vi "Global 2.vi"() -> ()   [LabVIEW 2018]
panel:
  in  "UsePython":bool caption="Tank RF"
  out "Fit OK":bool
  in  "Fupper":dbl=213.2 format="%#_13g"
  in  "Flower":dbl=212.8 format="%#_13g"
  in  "AutoFreq":bool
  in  "Tune file":string="Tune2.csv"
  out "Beam ON":bool=TRUE
  in  "NMR Channel":i32=2 min=0 max=7 step=1
  in  "TEQ Comment":string="Unused"
  in  "Q Comment":string="Newest  213 MHz Q curve 5/2/18"
  in  "TEQ file":string="NMRave.csv"
  in  "Measurement":enum16{"TEQ", "POL", "QCV"}(ring)=enum."QCV"
  in  "Commentary":string="Start trying python Q curve subtraction"
  in  "Calib Constant":dbl=1000.0 min=0.0 max=1000.0 step=0.001 format="%_3f"
  out "File name":string="C:\\users\\Ptgroup\\Desktop\\rssmt\\data\\22\\QCV3830786383.csv"
  in  "IP Address":string="192.168.24.146"
  in  "Gain":enum16{"LOW", "HI", "MAX"}(ring)
  in  "COM Port #":refnum<visa-resource-name>="COM8"
  out "Peak center (MHz)":sgl=212.9519 format="%.3f"
  in  "Logoffset (V)":dbl min=-9.0 max=0.0 step=0.0005 format="%_5g"
  in  "Phase (V)":dbl=2.566 min=-0.4 max=10.7 step=0.0005 format="%_5g"
  in  "Real/Quad Q curve":bool=TRUE
  out "Temperature (C)":dbl(graph)=24.75
  out "+3V supply":dbl=3.265 format="%_4g"
  out "Temp (C)":dbl=24.75 format="%_4g"
  in  "RemovePed":bool=TRUE
  in  "IF / LOG Det":bool=TRUE
  in  "Q curve file":string="QCV3608133393.csv"
  in  "AutoTune":bool
  out "RF OK":bool=TRUE
  out "Peak area (mV-MHz)":sgl=0.727321 format="%.3e"
  in  "Gauss Fit":bool
  out "NMR Graph + Fit":cluster{cluster{dbl, "Numeric":dbl}[]}[](graph)=[{[{224.27, "Numeric"=0.0}, {224.2705, "Numeric"=0.0}, {224.27100000000002, "Numeric"=0.0}, {224.2715, "Numeric"=0.0}, {224.27200000000002, "Numeric"=0.0}, {224.2725, "Numeric"=0.0}, {224.273, "Numeric"=0.0}, {224.2735, "Numeric"=0.0}, {224.274, "Numeric"=0.0}, {224.27450000000002, "Numeric"=0.0}, {224.275, "Numeric"=0.0}, {224.27550000000002, "Numeric"=0.0}, {224.276, "Numeric"=0.0}, {224.2765, "Numeric"=0.0}, {224.27700000000002, "Numeric"=0.0}, {224.2775, "Numeric"=0.0}, {224.27800000000002, "Numeric"=0.0}, {224.2785, "Numeric"=0.0}, {224.279, "Numeric"=0.0}, {224.2795, "Numeric"=0.0}, {224.28, "Numeric"=0.0}, {224.28050000000002, "Numeric"=0.0}, {224.281, "Numeric"=0.0}, {224.28150000000002, "Numeric"=0.0}, {224.282, "Numeric"=0.0}, {224.2825, "Numeric"=0.0}, {224.28300000000002, "Numeric"=0.0}, {224.2835, "Numeric"=0.0}, {224.28400000000002, "Numeric"=0.0}, {224.2845, "Numeric"=0.0}, {224.285, "Numeric"=0.0}, {224.2855, "Numeric"=0.0}, {224.286, "Numeric"=0.0}, {224.28650000000002, "Numeric"=0.0}, {224.287, "Numeric"=0.0}, {224.28750000000002, "Numeric"=0.0}, {224.288, "Numeric"=0.0}, {224.2885, "Numeric"=0.0}, {224.28900000000002, "Numeric"=0.0}, {224.2895, "Numeric"=0.0}, {224.29000000000002, "Numeric"=0.0}, {224.2905, "Numeric"=0.0}, {224.291, "Numeric"=0.0}, {224.2915, "Numeric"=0.0}, {224.292, "Numeric"=0.0}, {224.29250000000002, "Numeric"=0.0}, {224.293, "Numeric"=0.0}, {224.29350000000002, "Numeric"=0.0}, {224.294, "Numeric"=0.0}, {224.2945, "Numeric"=0.0}, {224.29500000000002, "Numeric"=0.0}, {224.2955, "Numeric"=0.0}, {224.29600000000002, "Numeric"=0.0}, {224.2965, "Numeric"=0.0}, {224.297, "Numeric"=0.0}, {224.2975, "Numeric"=0.0}, {224.298, "Numeric"=0.0}, {224.29850000000002, "Numeric"=0.0}, {224.299, "Numeric"=0.0}, {224.2995, "Numeric"=0.0}, {224.3, "Numeric"=0.0}, {224.3005, "Numeric"=0.0}, {224.30100000000002, "Numeric"=0.0}, {224.3015, "Numeric"=0.0}, {224.30200000000002, "Numeric"=0.0}, {224.3025, "Numeric"=0.0}, {224.303, "Numeric"=0.0}, {224.3035, "Numeric"=0.0}, {224.304, "Numeric"=0.0}, {224.30450000000002, "Numeric"=0.0}, {224.305, "Numeric"=0.0}, {224.3055, "Numeric"=0.0}, {224.306, "Numeric"=0.0}, {224.3065, "Numeric"=0.0}, {224.30700000000002, "Numeric"=0.0}, {224.3075, "Numeric"=0.0}, {224.30800000000002, "Numeric"=0.0}, {224.3085, "Numeric"=0.0}, {224.309, "Numeric"=0.0}, {224.3095, "Numeric"=0.0}, {224.31, "Numeric"=0.0}, {224.31050000000002, "Numeric"=0.0}, {224.311, "Numeric"=0.0}, {224.3115, "Numeric"=0.0}, {224.312, "Numeric"=0.0}, {224.3125, "Numeric"=0.0}, {224.31300000000002, "Numeric"=0.0}, {224.3135, "Numeric"=0.0}, {224.31400000000002, "Numeric"=0.0}, {224.3145, "Numeric"=0.0}, {224.315, "Numeric"=0.0}, {224.31550000000001, "Numeric"=0.0}, {224.316, "Numeric"=0.0}, {224.31650000000002, "Numeric"=0.0}, {224.317, "Numeric"=0.0}, {224.3175, "Numeric"=0.0}, {224.318, "Numeric"=0.0}, {224.3185, "Numeric"=0.0}, {224.31900000000002, "Numeric"=0.0}, {224.3195, "Numeric"=0.0}, {224.32, "Numeric"=0.0}, {224.3205, "Numeric"=0.0}, {224.321, "Numeric"=0.0}, {224.32150000000001, "Numeric"=0.0}, {224.322, "Numeric"=0.0}, {224.32250000000002, "Numeric"=0.0}, {224.323, "Numeric"=0.0}, {224.3235, "Numeric"=0.0}, {224.324, "Numeric"=0.0}, {224.3245, "Numeric"=0.0}, {224.32500000000002, "Numeric"=0.0}, {224.3255, "Numeric"=0.0}, {224.326, "Numeric"=0.0}, {224.3265, "Numeric"=0.0}, {224.327, "Numeric"=0.0}, {224.32750000000001, "Numeric"=0.0}, {224.328, "Numeric"=0.0}, {224.32850000000002, "Numeric"=0.0}, {224.329, "Numeric"=0.0}, {224.3295, "Numeric"=0.0}, {224.33, "Numeric"=0.0}, {224.3305, "Numeric"=0.0}, {224.33100000000002, "Numeric"=0.0}, {224.3315, "Numeric"=0.0}, {224.332, "Numeric"=0.0}, {224.3325, "Numeric"=0.0}, {224.333, "Numeric"=0.0}, {224.33350000000002, "Numeric"=0.0}, {224.334, "Numeric"=0.0}, {224.33450000000002, "Numeric"=0.0}, {224.335, "Numeric"=0.0}, {224.3355, "Numeric"=0.0}, {224.336, "Numeric"=0.0}, {224.3365, "Numeric"=0.0}, {224.33700000000002, "Numeric"=0.0}, {224.3375, "Numeric"=0.0}, {224.338, "Numeric"=0.0}, {224.3385, "Numeric"=0.0}, {224.339, "Numeric"=0.0}, {224.33950000000002, "Numeric"=0.0}, {224.34, "Numeric"=0.0}, {224.34050000000002, "Numeric"=0.0}, {224.341, "Numeric"=0.0}, {224.3415, "Numeric"=0.0}, {224.342, "Numeric"=0.0}, {224.3425, "Numeric"=0.0}, {224.34300000000002, "Numeric"=0.0}, {224.3435, "Numeric"=0.0}, {224.344, "Numeric"=0.0}, {224.3445, "Numeric"=0.0}, {224.345, "Numeric"=0.0}, {224.34550000000002, "Numeric"=0.0}, {224.346, "Numeric"=0.0}, {224.3465, "Numeric"=0.0}, {224.347, "Numeric"=0.0}, {224.3475, "Numeric"=0.0}, {224.348, "Numeric"=0.0}, {224.3485, "Numeric"=0.0}, {224.34900000000002, "Numeric"=0.0}, {224.3495, "Numeric"=0.0}, {224.35, "Numeric"=0.0}, {224.3505, "Numeric"=0.0}, {224.351, "Numeric"=0.0}, {224.35150000000002, "Numeric"=0.0}, {224.352, "Numeric"=0.0}, {224.3525, "Numeric"=0.0}, {224.353, "Numeric"=0.0}, {224.3535, "Numeric"=0.0}, {224.354, "Numeric"=0.0}, {224.3545, "Numeric"=0.0}, {224.35500000000002, "Numeric"=0.0}, {224.3555, "Numeric"=0.0}, {224.356, "Numeric"=0.0}, {224.3565, "Numeric"=0.0}, {224.357, "Numeric"=0.0}, {224.35750000000002, "Numeric"=0.0}, {224.358, "Numeric"=0.0}, {224.3585, "Numeric"=0.0}, {224.359, "Numeric"=0.0}, {224.3595, "Numeric"=0.0}, {224.36, "Numeric"=0.0}, {224.3605, "Numeric"=0.0}, {224.36100000000002, "Numeric"=0.0}, {224.3615, "Numeric"=0.0}, {224.362, "Numeric"=0.0}, {224.3625, "Numeric"=0.0}, {224.363, "Numeric"=0.0}, {224.36350000000002, "Numeric"=0.0}, {224.364, "Numeric"=0.0}, {224.3645, "Numeric"=0.0}, {224.365, "Numeric"=0.0}, {224.3655, "Numeric"=0.0}, {224.366, "Numeric"=0.0}, {224.3665, "Numeric"=0.0}, {224.36700000000002, "Numeric"=0.0}, {224.3675, "Numeric"=0.0}, {224.368, "Numeric"=0.0}, {224.3685, "Numeric"=0.0}, {224.369, "Numeric"=0.0}, {224.36950000000002, "Numeric"=0.0}, {224.37, "Numeric"=0.0}, {224.3705, "Numeric"=0.0}, {224.371, "Numeric"=0.0}, {224.3715, "Numeric"=0.0}, {224.372, "Numeric"=0.0}, {224.3725, "Numeric"=0.0}, {224.373, "Numeric"=0.0}, {224.3735, "Numeric"=0.0}, {224.374, "Numeric"=0.0}, {224.3745, "Numeric"=0.0}, {224.375, "Numeric"=0.0}, {224.37550000000002, "Numeric"=0.0}, {224.376, "Numeric"=0.0}, {224.3765, "Numeric"=0.0}, {224.377, "Numeric"=0.0}, {224.3775, "Numeric"=0.0}, {224.37800000000001, "Numeric"=0.0}, {224.3785, "Numeric"=0.0}, {224.379, "Numeric"=0.0}, {224.3795, "Numeric"=0.0}, {224.38, "Numeric"=0.0}, {224.3805, "Numeric"=0.0}, {224.381, "Numeric"=0.0}, {224.38150000000002, "Numeric"=0.0}, {224.382, "Numeric"=0.0}, {224.3825, "Numeric"=0.0}, {224.383, "Numeric"=0.0}, {224.3835, "Numeric"=0.0}, {224.38400000000001, "Numeric"=0.0}, {224.3845, "Numeric"=0.0}, {224.385, "Numeric"=0.0}, {224.3855, "Numeric"=0.0}, {224.386, "Numeric"=0.0}, {224.3865, "Numeric"=0.0}, {224.387, "Numeric"=0.0}, {224.38750000000002, "Numeric"=0.0}, {224.388, "Numeric"=0.0}, {224.3885, "Numeric"=0.0}, {224.389, "Numeric"=0.0}, {224.3895, "Numeric"=0.0}, {224.39000000000001, "Numeric"=0.0}, {224.3905, "Numeric"=0.0}, {224.391, "Numeric"=0.0}, {224.3915, "Numeric"=0.0}, {224.392, "Numeric"=0.0}, {224.3925, "Numeric"=0.0}, {224.393, "Numeric"=0.0}, {224.39350000000002, "Numeric"=0.0}, {224.394, "Numeric"=0.0}, {224.3945, "Numeric"=0.0}, {224.395, "Numeric"=0.0}, {224.3955, "Numeric"=0.0}, {224.39600000000002, "Numeric"=0.0}, {224.3965, "Numeric"=0.0}, {224.397, "Numeric"=0.0}, {224.3975, "Numeric"=0.0}, {224.398, "Numeric"=0.0}, {224.3985, "Numeric"=0.0}, {224.399, "Numeric"=0.0}, {224.3995, "Numeric"=0.0}, {224.4, "Numeric"=0.0}, {224.4005, "Numeric"=0.0}, {224.401, "Numeric"=0.0}, {224.4015, "Numeric"=0.0}, {224.40200000000002, "Numeric"=0.0}, {224.4025, "Numeric"=0.0}, {224.403, "Numeric"=0.0}, {224.4035, "Numeric"=0.0}, {224.404, "Numeric"=0.0}, {224.4045, "Numeric"=0.0}, {224.405, "Numeric"=0.0}, {224.4055, "Numeric"=0.0}, {224.406, "Numeric"=0.0}, {224.4065, "Numeric"=0.0}, {224.407, "Numeric"=0.0}, {224.4075, "Numeric"=0.0}, {224.40800000000002, "Numeric"=0.0}, {224.4085, "Numeric"=0.0}, {224.409, "Numeric"=0.0}, {224.4095, "Numeric"=0.0}, {224.41, "Numeric"=0.0}, {224.4105, "Numeric"=0.0}, {224.411, "Numeric"=0.0}, {224.4115, "Numeric"=0.0}, {224.412, "Numeric"=0.0}, {224.4125, "Numeric"=0.0}, {224.413, "Numeric"=0.0}, {224.4135, "Numeric"=0.0}, {224.41400000000002, "Numeric"=0.0}, {224.4145, "Numeric"=0.0}, {224.415, "Numeric"=0.0}, {224.4155, "Numeric"=0.0}, {224.416, "Numeric"=0.0}, {224.4165, "Numeric"=0.0}, {224.417, "Numeric"=0.0}, {224.4175, "Numeric"=0.0}, {224.418, "Numeric"=0.0}, {224.4185, "Numeric"=0.0}, {224.419, "Numeric"=0.0}, {224.4195, "Numeric"=0.0}, {224.42000000000002, "Numeric"=0.0}, {224.4205, "Numeric"=0.0}, {224.421, "Numeric"=0.0}, {224.4215, "Numeric"=0.0}, {224.422, "Numeric"=0.0}, {224.4225, "Numeric"=0.0}, {224.423, "Numeric"=0.0}, {224.4235, "Numeric"=0.0}, {224.424, "Numeric"=0.0}, {224.4245, "Numeric"=0.0}, {224.425, "Numeric"=0.0}, {224.4255, "Numeric"=0.0}, {224.426, "Numeric"=0.0}, {224.4265, "Numeric"=0.0}, {224.427, "Numeric"=0.0}, {224.4275, "Numeric"=0.0}, {224.428, "Numeric"=0.0}, {224.4285, "Numeric"=0.0}, {224.429, "Numeric"=0.0}, {224.4295, "Numeric"=0.0}, {224.43, "Numeric"=0.0}, {224.4305, "Numeric"=0.0}, {224.431, "Numeric"=0.0}, {224.4315, "Numeric"=0.0}, {224.432, "Numeric"=0.0}, {224.4325, "Numeric"=0.0}, {224.433, "Numeric"=0.0}, {224.4335, "Numeric"=0.0}, {224.434, "Numeric"=0.0}, {224.4345, "Numeric"=0.0}, {224.435, "Numeric"=0.0}, {224.4355, "Numeric"=0.0}, {224.436, "Numeric"=0.0}, {224.4365, "Numeric"=0.0}, {224.437, "Numeric"=0.0}, {224.4375, "Numeric"=0.0}, {224.438, "Numeric"=0.0}, {224.4385, "Numeric"=0.0}, {224.439, "Numeric"=0.0}, {224.4395, "Numeric"=0.0}, {224.44, "Numeric"=0.0}, {224.44050000000001, "Numeric"=0.0}, {224.441, "Numeric"=0.0}, {224.4415, "Numeric"=0.0}, {224.442, "Numeric"=0.0}, {224.4425, "Numeric"=0.0}, {224.443, "Numeric"=0.0}, {224.4435, "Numeric"=0.0}, {224.444, "Numeric"=0.0}, {224.4445, "Numeric"=0.0}, {224.445, "Numeric"=0.0}, {224.4455, "Numeric"=0.0}, {224.446, "Numeric"=0.0}, {224.4465, "Numeric"=0.0}, {224.447, "Numeric"=0.0}, {224.4475, "Numeric"=0.0}, {224.448, "Numeric"=0.0}, {224.4485, "Numeric"=0.0}, {224.449, "Numeric"=0.0}, {224.4495, "Numeric"=0.0}, {224.45, "Numeric"=0.0}, {224.4505, "Numeric"=0.0}, {224.451, "Numeric"=0.0}, {224.4515, "Numeric"=0.0}, {224.452, "Numeric"=0.0}, {224.4525, "Numeric"=0.0}, {224.453, "Numeric"=0.0}, {224.4535, "Numeric"=0.0}, {224.454, "Numeric"=0.0}, {224.4545, "Numeric"=0.0}, {224.455, "Numeric"=0.0}, {224.4555, "Numeric"=0.0}, {224.456, "Numeric"=0.0}, {224.4565, "Numeric"=0.0}, {224.457, "Numeric"=0.0}, {224.4575, "Numeric"=0.0}, {224.458, "Numeric"=0.0}, {224.4585, "Numeric"=0.0}, {224.459, "Numeric"=0.0}, {224.4595, "Numeric"=0.0}, {224.46, "Numeric"=0.0}, {224.4605, "Numeric"=0.0}, {224.461, "Numeric"=0.0}, {224.4615, "Numeric"=0.0}, {224.462, "Numeric"=0.0}, {224.4625, "Numeric"=0.0}, {224.463, "Numeric"=0.0}, {224.4635, "Numeric"=0.0}, {224.464, "Numeric"=0.0}, {224.4645, "Numeric"=0.0}, {224.465, "Numeric"=0.0}, {224.4655, "Numeric"=0.0}, {224.466, "Numeric"=0.0}, {224.4665, "Numeric"=0.0}, {224.467, "Numeric"=0.0}, {224.4675, "Numeric"=0.0}, {224.468, "Numeric"=0.0}, {224.4685, "Numeric"=0.0}, {224.469, "Numeric"=0.0}, {224.4695, "Numeric"=0.0}, {224.47, "Numeric"=0.0}]}]
  in  "Amp of Q curve":dbl=0.8 min=-1000.0 max=1000.0 step=0.01 format="%_3f"
  in  "Subtract Q curve":bool
  out "Pedestal Offset":dbl(graph)=4.999847412109375
  out "Pedestal Difference":dbl(graph)=-0.0
  out "# Good Spectra":i32=497
  in  "Quality cuts":bool=TRUE
  out "Pedestal OK":bool=TRUE
  out "Sweep #":i32=47
  out "1st Sweep":bool
  out "ADC volts OK":bool
  out "Peak Height Distribution":cluster{"Y":dbl[], "Y":dbl[]}[](graph)=[{"Y"=[13.230458907623072, 13.230965880889674, 13.231472854156275, 13.231979827422876, 13.232486800689477, 13.23299377395608, 13.233500747222681, 13.234007720489283, 13.234514693755884, 13.235021667022485, 13.235528640289088, 13.23603561355569, 13.23654258682229, 13.237049560088892, 13.237556533355495, 13.238063506622096, 13.238570479888697, 13.239077453155298, 13.2395844264219, 13.240091399688502, 13.240598372955104, 13.241105346221705, 13.241612319488306, 13.242119292754907, 13.24262626602151, 13.243133239288111, 13.243640212554713, 13.244147185821314, 13.244654159087915, 13.245161132354518, 13.24566810562112, 13.24617507888772, 13.246682052154322, 13.247189025420925, 13.247695998687526, 13.248202971954127, 13.248709945220728, 13.24921691848733, 13.249723891753932, 13.250230865020534, 13.250737838287135, 13.251244811553736, 13.251751784820337, 13.25225875808694, 13.252765731353541, 13.253272704620143, 13.253779677886744, 13.254286651153345, 13.254793624419948, 13.25530059768655, 13.25580757095315, 13.256314544219752, 13.256821517486355, 13.257328490752956, 13.257835464019557, 13.258342437286158, 13.25884941055276, 13.259356383819362, 13.259863357085964, 13.260370330352565, 13.260877303619166, 13.261384276885767, 13.26189125015237, 13.262398223418971, 13.262905196685573, 13.263412169952174, 13.263919143218775, 13.264426116485378, 13.26493308975198, 13.26544006301858, 13.265947036285182, 13.266454009551785, 13.266960982818386, 13.267467956084987, 13.267974929351588, 13.26848190261819, 13.268988875884792, 13.269495849151394, 13.270002822417995, 13.270509795684596, 13.271016768951197, 13.2715237422178, 13.272030715484401, 13.272537688751003, 13.273044662017604, 13.273551635284205, 13.274058608550808, 13.27456558181741, 13.27507255508401, 13.275579528350612, 13.276086501617215, 13.276593474883816, 13.277100448150417, 13.277607421417018, 13.27811439468362, 13.278621367950223, 13.279128341216824, 13.279635314483425, 13.280142287750026, 13.280649261016627], "Y"=[1.0, 0.0, 0.0, 0.0, 0.0, 0.0, 0.0, 0.0, 0.0, 0.0, 0.0, 0.0, 1.0, 1.0, 0.0, 2.0, 2.0, 2.0, 1.0, 5.0, 2.0, 3.0, 3.0, 3.0, 4.0, 3.0, 5.0, 4.0, 8.0, 7.0, 4.0, 10.0, 8.0, 7.0, 5.0, 6.0, 8.0, 4.0, 8.0, 11.0, 8.0, 6.0, 13.0, 10.0, 5.0, 12.0, 7.0, 11.0, 15.0, 13.0, 4.0, 14.0, 12.0, 12.0, 10.0, 10.0, 10.0, 7.0, 9.0, 12.0, 6.0, 8.0, 5.0, 6.0, 7.0, 10.0, 8.0, 3.0, 7.0, 11.0, 5.0, 7.0, 7.0, 5.0, 5.0, 7.0, 5.0, 2.0, 2.0, 4.0, 4.0, 9.0, 4.0, 2.0, 2.0, 4.0, 2.0, 0.0, 3.0, 3.0, 2.0, 1.0, 3.0, 1.0, 1.0, 1.0, 1.0, 1.0, 3.0, 2.0]}]
  in  "# of Sweeps":i32=500
  out "S/N":dbl=1383.7970737015771 format="%_3g"
  out "Peak mean (V)":dbl=13.257193605897562 format="%_4g"
  out "Peak Height":dbl(graph)=0.7273210385932467
  in  "Raw Data":bool=TRUE
  in  "Tank RF":bool
  out "IF Atten (dB)":i8=7 min=0 max=31 step=1
  in  "IFoffset (V)":dbl=4.4757 min=-9.0 max=9.0 step=0.001 format="%.4f"
  in  "Tune  (V)":dbl=0.18499999999999925 min=-0.5 max=8.0 step=0.001 format="%.4f"
  in  "Invert Polarity":bool
  out "Pedestal Diff (V)":sgl=-0.0 format="%.3f"
  out "Peak amp (V)":sgl format="%.4f"
  in  "Save Data to File":bool=TRUE
  out "RF Level (dBm)":dbl=4.0 min=-10.0 max=10.0 step=0.1 format="%.2f"
  out "Sample RMS (V)":dbl format="%.4f"
  in  "# Sample/step":i32=20 min=1 max=1000 step=1
  in  "Step Width (MHz)":dbl=0.002 min=0.0 max=1000.0 step=1e-05 format="%.5f"
  in  "Freq Span (MHz)":dbl=0.8 min=0.0 max=50.0 step=0.1 format="%.3f"
  in  "Center Freq (MHz)":dbl=213.0 min=20.0 max=300.0 step=0.1 format="%.3f"
  # "Settings"
  # "E1039 Global NMR Control Panel"
  # "R\nF\n\nG\nE\nN \n\n+\n\nI\nF"
  # "D\nA\nC\ns"
  # "A\nD\nC"
  # "I\n/\nO"
  # "D\nA\nT\nA\n\nA \nN\nA\nL\nY\nS\nI\nS"
  # "Qcurve"
  # "Quad"
  # "Quad"
  # "Integral Area"
  # "Polarization"
  # "/ Integral Area"
  # "Results"
  # "A\nv\ne\nr\na\ng\ne\ns"
  # "S\nw\ne\ne\np"
  # "Q Curve subtraction limits"
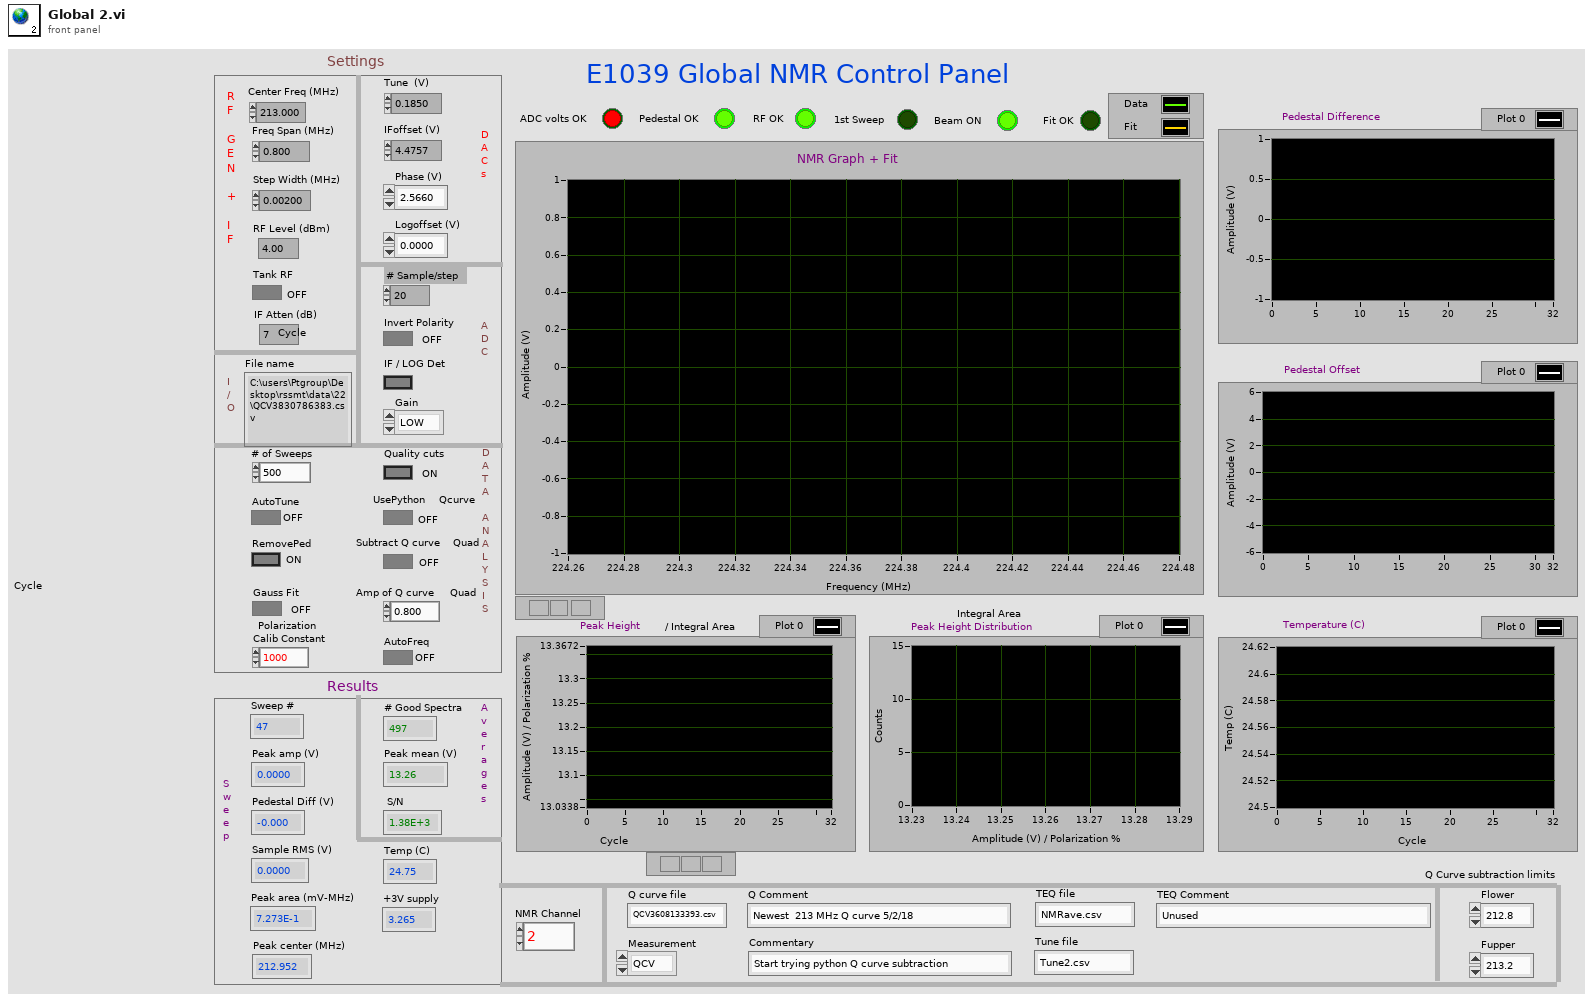
[diagram p1: front panel]
diagram:
